vi "DAQ- Steper.vi"(0 "Travel (Degree)":dbl=100.0, 1 "Mode":i32(ring)=10178 items=["Finite Samples"=10178, "Continuous Samples"=10123, "Hardware Timed Single Point"=12522], 5 "Home Condition":bool, 7 "Speed d/s":dbl=10.0, 11 "error in":errorcluster) -> (4 "Task Done Bit":bool, 14 "error out":errorcluster)   [LabVIEW 2015]
uses:
  Project Setup/Globle Variable/GR_Servo.vi
  Galobal variable_TI.vi
  <vilib>/DAQmx/create/channels.llb/DAQmx Create Channel (CO-Pulse Generation-Frequency).vi
  <vilib>/DAQmx/configure/timing.llb/DAQmx Timing (Implicit).vi
panel:
  in  "Motor PPR":dbl=3600.0
  in  "Motor Gear Ratio":dbl=1.0
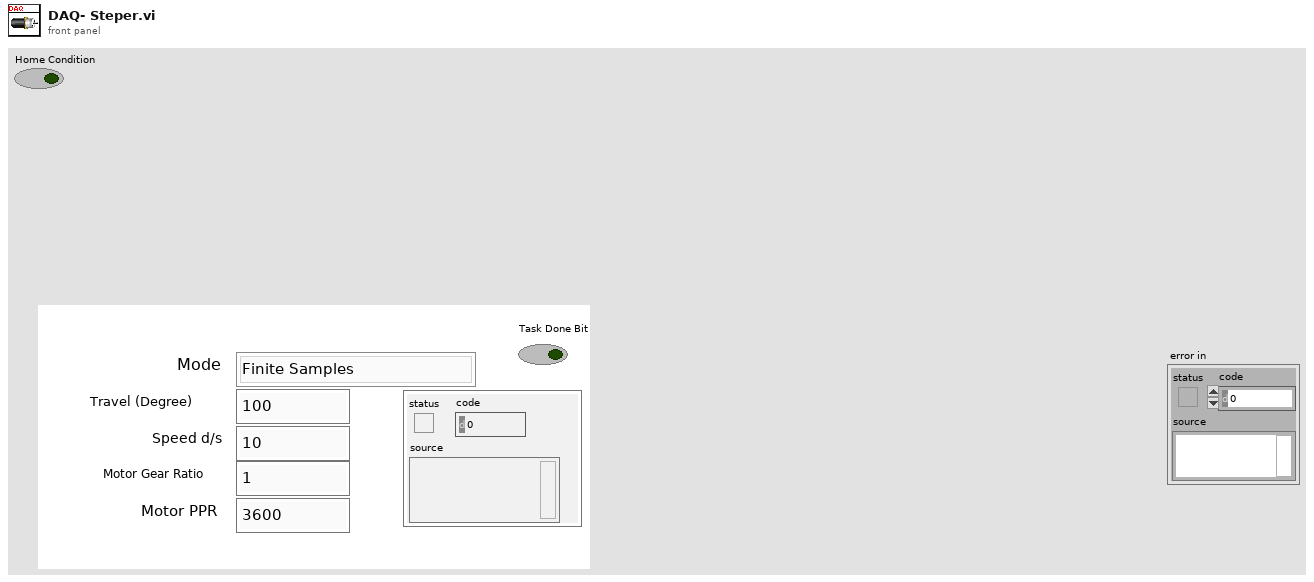
[diagram p1: front panel]
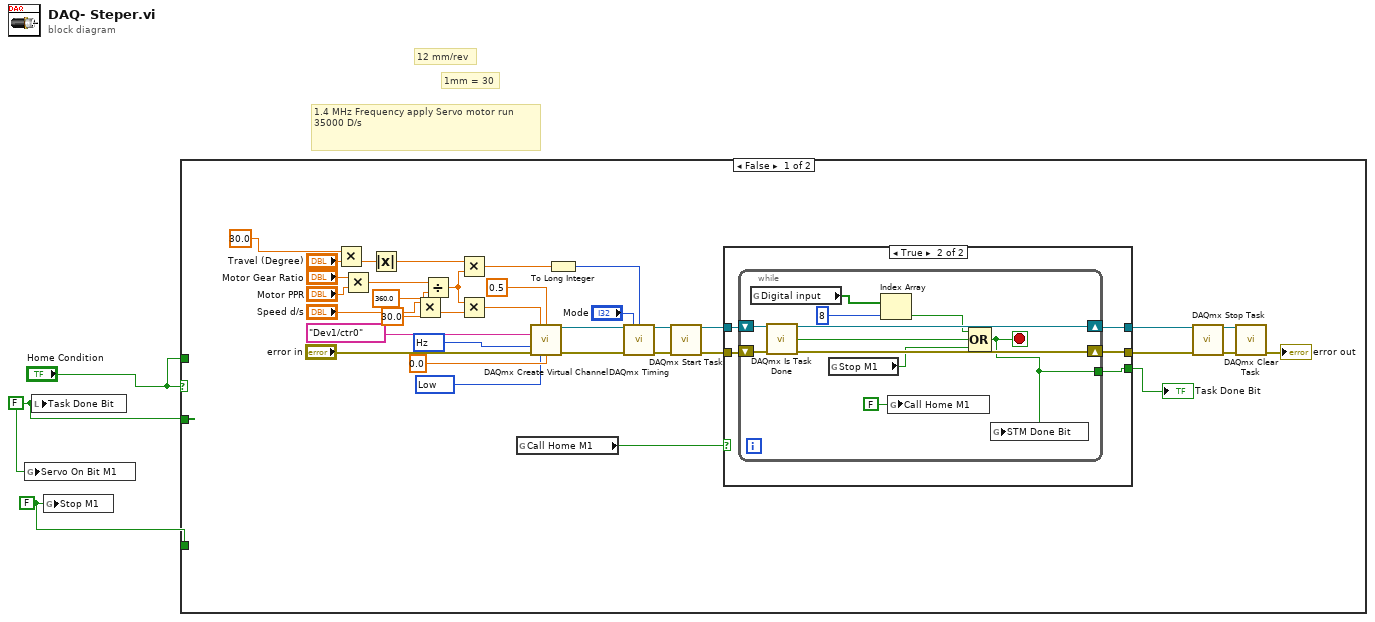
[diagram p0: block diagram]
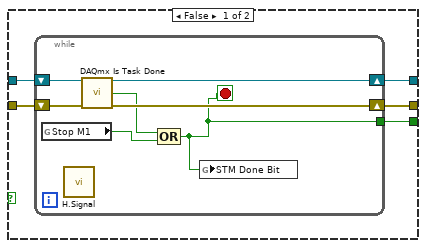
[diagram p2: hidden frame]
diagram:
  w2 = FALSE ("Stop M1")
  w3 = FALSE ("Task Done Bit")
  # "1mm = 30"
  # "12 mm/rev"
  # "1.4 MHz Frequency apply Servo motor run \n35000 D/s"
  n1 = global write "GR_Servo.vi" "Servo On Bit M1"(w3) -> ()
  n2 = local write "Task Done Bit"(w3) -> ()
  n3 = global write "Galobal variable_TI.vi" "Stop M1"(w2) -> ()
  n4 = case shown="False" "Home Condition" {
    tunnel: w3 -> [_ _]
    tunnel: w2 -> [_ _]
    tunnel: "Home Condition" -> [_ _]
    frame False {
      w14 = 10373 items=["Hz"=10373] ("units")
      w15 = 10214 items=["High"=10192, "Low"=10214] ("idle state")
      n5 = Multiply(x=30.0, y="Travel (Degree)") -> (x*y=w10:dbl)
      n6 = Multiply(x="Motor Gear Ratio", y="Motor PPR") -> (x*y=w24:dbl)
      n7 = Absolute Value(x=w10) -> (abs(x)=w23:dbl)
      n8 = Multiply(x="Speed d/s", y=30.0) -> (x*y=w8:dbl)
      n9 = Divide(x=w24, y=360.0) -> (x/y=w30:dbl)
      n10 = Multiply(x=w23, y=w30) -> (x*y=w28:dbl)
      n11 = Multiply(x=w30, y=w8) -> (x*y=w35:dbl)
      n12 = global read "Galobal variable_TI.vi" "Call Home M1"() -> (w5:bool)
      n13 = call-poly <vilib>:"DAQmx Create Virtual Channel.vi"("frequency"=w35, "duty cycle"=0.5, "counter"=tag "Dev1/ctr0", "units"=w14, "error in"="error in", "idle state"=w15, "initial delay"=0.0) -> ("task out"=w17:refnum<k21>, "error out"=w18:errorcluster)  [unwired: 7 in]
      n14 = To Long Integer(number=w28) -> (32bit integer=w38:i32)
      n15 = call-poly <vilib>:"DAQmx Timing.vi"("task/channels in"=w17, "sample mode"="Mode", "samples per channel"=w38, "error in"=w18) -> ("task out"=w19:refnum<k21>, "error out"=w20:errorcluster)  [unwired: 10 in]
      n16 = call <vilib>:"DAQmx Start Task.vi"("task/channels in"=w19, "error in"=w20) -> ("task out"=w13:refnum<k21>, "error out"=w11:errorcluster)  [unwired: 12 in]
      n17 = case shown="True" w5 {
        tunnel: [w43 w52] -> w33
        tunnel: w13 -> [w42 w55]
        tunnel: [w41 w53] -> w12
        tunnel: w11 -> [w40 w54]
        tunnel: [w39 w51] -> w4
        frame False {
          n18 = while {
            shift-right: [w48] -> w41
            shift-left: w42 -> [w50]
            shift-right: [w49] -> w43
            shift-left: w40 -> [w47]
            tunnel: [w44] -> w39
            stop <- w44 stop-if-true
            n19 = global read "Galobal variable_TI.vi" "Stop M1"() -> (w45:bool)
            n20 = call "H.Signal.vi"() -> ()  [unwired: 11 in, 5 out]
            n21 = call <vilib>:"DAQmx Is Task Done.vi"("task/channels in"=w50, "error in"=w47) -> ("task out"=w48:refnum<k21>, "task done?"=w46:bool, "error out"=w49:errorcluster)  [unwired: 11 in]
            n22 = Compound Arithmetic op=OR(w46, w45) -> (w44:bool)
            n23 = global write "Galobal variable_TI.vi" "STM Done Bit"(w44) -> ()
          }
        }
        frame True {
          n24 = while {
            shift-right: [w64] -> w53
            shift-left: w55 -> [w66]
            shift-right: [w65] -> w52
            shift-left: w54 -> [w63]
            tunnel: [w57] -> w51
            stop <- w57 stop-if-true
            n25 = global read "Galobal variable_TI.vi" "Digital input"() -> (w59:bool[])
            n26 = call <vilib>:"DAQmx Is Task Done.vi"("task/channels in"=w66, "error in"=w63) -> ("task out"=w64:refnum<k21>, "task done?"=w62:bool, "error out"=w65:errorcluster)  [unwired: 11 in]
            n27 = global read "Galobal variable_TI.vi" "Stop M1"() -> (w61:bool)
            n28 = Index Array(array=w59, index=8) -> (element=w58:bool)
            n29 = global write "Galobal variable_TI.vi" "Call Home M1"(FALSE ("Call Home M1")) -> ()
            n30 = Compound Arithmetic op=OR(w58, w62, w61) -> (w57:bool)
            n31 = global write "Galobal variable_TI.vi" "STM Done Bit"(w57) -> ()
          }
        }
      }
      "Task Done Bit" <- w4
      n32 = call <vilib>:"DAQmx Stop Task.vi"("task/channels in"=w12, "error in"=w33) -> ("task out"=w21:refnum<k21>, "error out"=w34:errorcluster)  [unwired: 12 in]
      n33 = call <vilib>:"DAQmx Clear Task.vi"("task in"=w21, "error in"=w34) -> ("error out"=→"error out":errorcluster)  [unwired: 13 in]
    }
    frame True {
    }
  }
